vi "Prova QH.vi"(4 "solo acquisizione!!":bool=TRUE, 6 "Text.Text":string="Prova QH: ", 7 "Tipo motore pompa":enum16{"Monofase", "Trifase"}(ring), 8 "Array % valvole":dbl[][](array[numeric]), 9 "Manuale F\\auto T":bool=TRUE, 10 "Status":refnum<vi>, 11 "input cluster":T1={"Scelta wattmetro"={"Wattmetro"=enum."No Selection"}, "SET RPM"=0.0, "SET TEMP"=0.0, "Array banchi"=[{"Nome"="Elettropompa", "Tors. scala1"=0, "Tors. scala2"=0, "rpm"=0, "TAMB"=0, "Indici Temperature"=[0, 1], "Indice freno"=1, "alimentatore trifase"=0, "alimentatore monofase"=0, "alimentatore dc arm"=0, "alimentatore dc ecc"=0, "alimentatore dc mp"=0}, {"Nome"="Sommersa", "Tors. scala1"=0, "Tors. scala2"=0, "rpm"=0, "TAMB"=1, "Indici Temperature"=[0, 1], "Indice freno"=0, "alimentatore trifase"=0, "alimentatore monofase"=0, "alimentatore dc arm"=0, "alimentatore dc ecc"=0, "alimentatore dc mp"=0}], "Array valvole linee avvio/fermata"=[], "banco selezionato"=0, "Nomi valvole prop sistema"=[], "canale-- sensore"=[], "Attriti B1"=[], "Attriti B2"=[], "Collegamento elettrico"={"ALIMENTAZIONE ELETTRICA"=enum."AC MONOFASE", "ID"=0, "#rami freddo\\eq term resmeter"=0, "#rami riscaldamento resmeter"=0, "#rami freddo\\eq term resistomat"=0, "#rami riscaldamento resistomat"=0, "CALCOLI"=enum."AC TRIFASE"}, "lingua"=0, "Costanti collaudo"={"P [bar]"=0.0, "T amb. [°C]"=0.0, "Umidità [%]"=0.0, "T acqua [°C] 2"=0.0}, "OPZIONI MISURE RES"={"MISURA A FREDDO"=enum."RESISTOMAT", "MISURA EQ. TERMICO"=enum."RESISTOMAT", "MISURA DT PROVA IN CORSO"=enum."RESISTOMAT - CON FERMATE", "MISURE PRIMA E DOPO"=enum."RESISTOMAT", "STRUMENTI PRESENTI"=enum."NESSUNO"}, "Dati targa motore"={"Vnom"=0.0, "Fnom"=0.0, "Inom"=0.0, "Cnom"=0.0, "Npoli"=0.0, "Scorta 1"=0.0, "Scorta 2"=0.0, "Scorta 3"=0.0}}) -> ()   [LabVIEW 2019]
uses:
  Tstabilizzazione auto.vi
  SubVI ELETTROTEST60A Folder/Elettrotest60A/Global_bypass_ResMeter.vi
  TypeDef/WT SELECTION.ctl
  TypeDef/Definizione linea.ctl
  TypeDef/Cluster INFO.ctl
  TypeDef/Collegamenti_elettrici.ctl
  TypeDef/Control Calcoli.ctl
panel:
  out "Fine acq":bool
  in  "Reset":bool
  out "Set% valvole":dbl[](array[numeric])
  in  "Stato auto":string
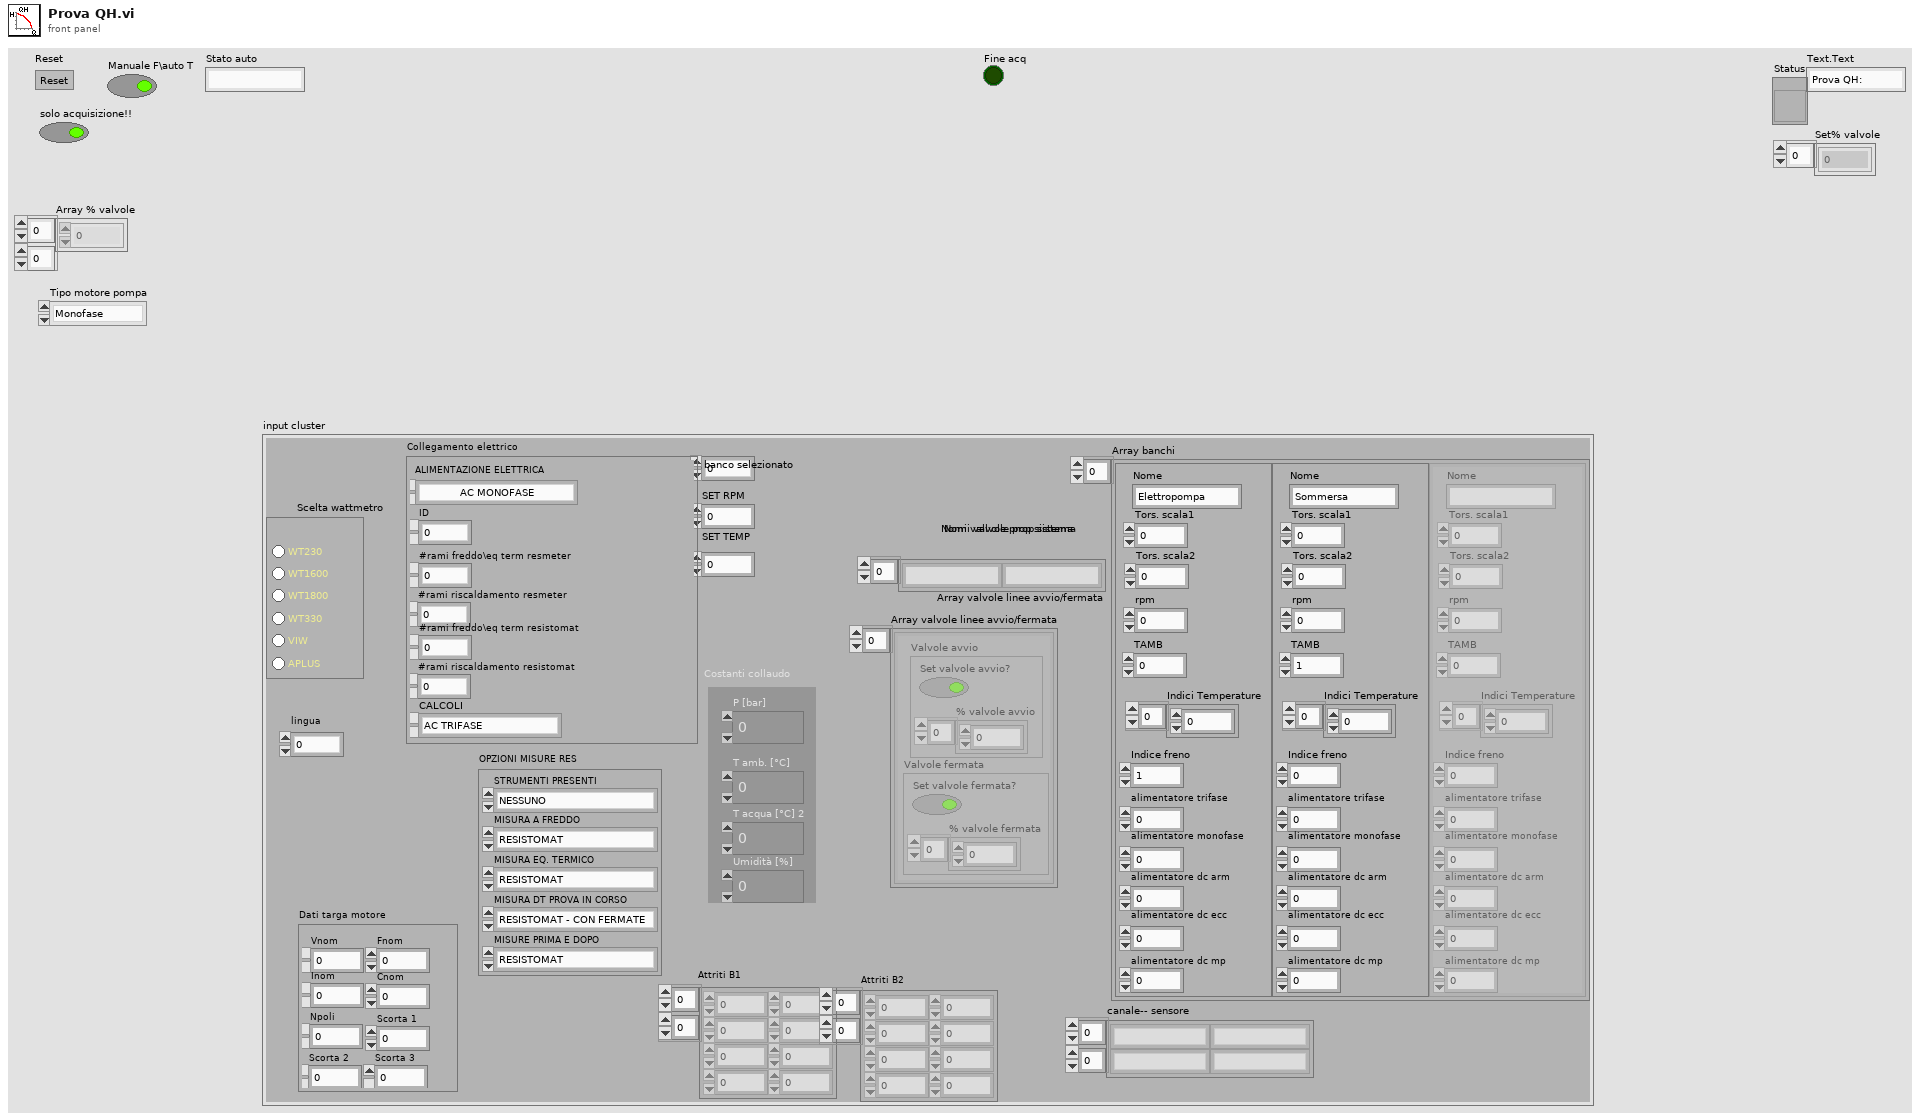
[diagram p1: front panel]
types:
  T1 = typedef "Cluster INFO.ctl" = cluster{"Scelta wattmetro":cluster{"Wattmetro":T2}, "SET RPM":dbl, "SET TEMP":dbl, "Array banchi":T3[], "Array valvole linee avvio/fermata":cluster{"Valvole avvio":cluster{"Set valvole avvio?":bool, "% valvole avvio":dbl[]}, "Valvole fermata":cluster{"Set valvole fermata?":bool, "% valvole fermata":dbl[]}}[], "banco selezionato":i8, "Nomi valvole prop sistema":string[], "canale-- sensore":string[][], "Attriti B1":dbl[][], "Attriti B2":dbl[][], "Collegamento elettrico":cluster{"ALIMENTAZIONE ELETTRICA":T4, "ID":i16, "#rami freddo\\eq term resmeter":i16, "#rami riscaldamento resmeter":i16, "#rami freddo\\eq term resistomat":i16, "#rami riscaldamento resistomat":i16, "CALCOLI":T5}, "lingua":i16, "Costanti collaudo":cluster{"P [bar]":dbl, "T amb. [°C]":dbl, "Umidità [%]":dbl, "T acqua [°C] 2":dbl}, "OPZIONI MISURE RES":cluster{"MISURA A FREDDO":enum16{"NESSUNO", "RESISTOMAT", "RES METER", "ENTRAMBI"}, "MISURA EQ. TERMICO":enum16{"NESSUNO", "RESISTOMAT", "RES METER", "ENTRAMBI"}, "MISURA DT PROVA IN CORSO":enum16{"NESSUNO", "RESISTOMAT - CON FERMATE", "RES METER - CON FERMATE", "RES METER - CONTINUO"}, "MISURE PRIMA E DOPO":enum16{"NESSUNO", "RESISTOMAT", "RES METER"}, "STRUMENTI PRESENTI":enum16{"NESSUNO", "RESISTOMAT", "RES METER", "ENTRAMBI"}}, "Dati targa motore":cluster{"Vnom":dbl, "Fnom":dbl, "Inom":dbl, "Cnom":dbl, "Npoli":dbl, "Scorta 1":dbl, "Scorta 2":dbl, "Scorta 3":dbl}}
  T2 = typedef "WT SELECTION.ctl" = enum32{"No Selection", "WT230", "WT1600", "WT1800", "WT330", "VIW", "APLUS"}
  T3 = typedef "Definizione linea.ctl" = cluster{"Nome":string, "Tors. scala1":i32, "Tors. scala2":i32, "rpm":i32, "TAMB":i32, "Indici Temperature":i16[], "Indice freno":i16, "alimentatore trifase":i16, "alimentatore monofase":i16, "alimentatore dc arm":i16, "alimentatore dc ecc":i16, "alimentatore dc mp":i16}
  T4 = typedef "Collegamenti_elettrici.ctl" = enum16{"AC TRIFASE", "AC TRIFASE + FRENO", "AC MONOFASE", "DC CON ECCITAZIONE", "DC CON ECCITAZIONE + FRENO", "DC NO ECCITAZIONE", "DC NO ECCITAZIONE + FRENO", "FRENO TRASC + AFE", "SOLO FRENO", "CARICO RESISTIVO", "GENERICO", "SOLO ACQUISITORE", "SCORTA 4", "SCORTA 5", "SCORTA 6"}
  T5 = typedef "Control Calcoli.ctl" = enum16{"AC TRIFASE", "AC MONOFASE", "DC ECCITAZIONE", "DC NO ECCITAZIONE", "POMPA TRIFASE", "POMPA MONOFASE", "GENERICO", "TRASFORMATORE", "ALTERNATORE TRASCINATO", "GRUPPO ELETTROGENO"}
  T6 = cluster{"Valvole avvio":cluster{"Set valvole avvio?":bool, "% valvole avvio":dbl[]}, "Valvole fermata":cluster{"Set valvole fermata?":bool, "% valvole fermata":dbl[]}}[]
  T7 = cluster{"Valvole avvio":cluster{"Set valvole avvio?":bool, "% valvole avvio":dbl[]}, "Valvole fermata":cluster{"Set valvole fermata?":bool, "% valvole fermata":dbl[]}}
  T8 = cluster{"Set valvole avvio?":bool, "% valvole avvio":dbl[]}
  T9 = cluster{"Set valvole fermata?":bool, "% valvole fermata":dbl[]}
  T10 = cluster{"Array of elements":cluster{"String":string, "variant":variant}[], "Single element":cluster{"String":string, "variant":variant}, "enque at\nopposite end (F)":bool, "no replications (F)":bool}
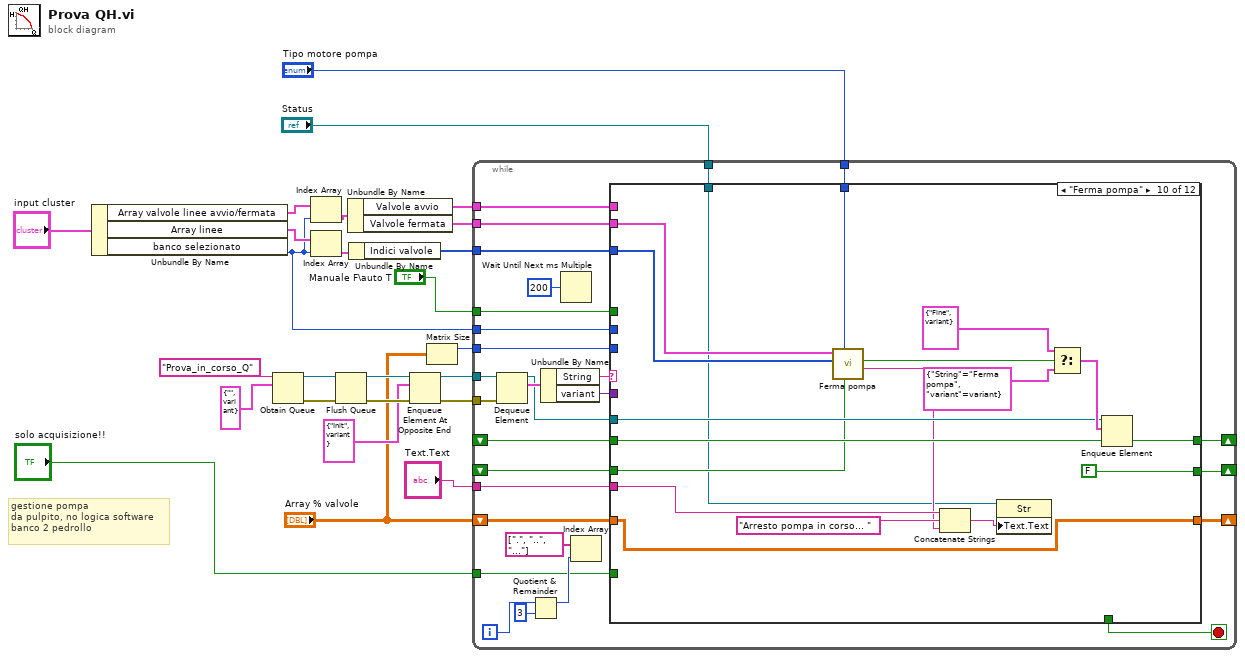
[diagram p0: block diagram]
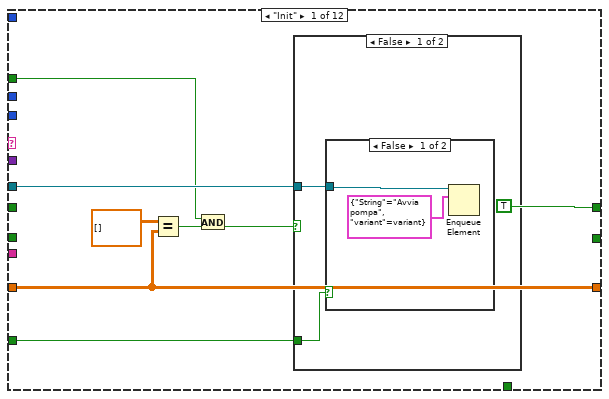
[diagram p2: hidden frame]
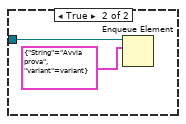
[diagram p3: hidden frame]
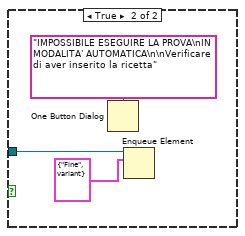
[diagram p4: hidden frame]
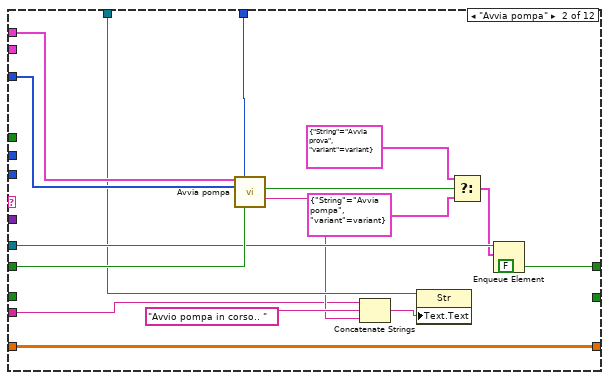
[diagram p5: hidden frame]
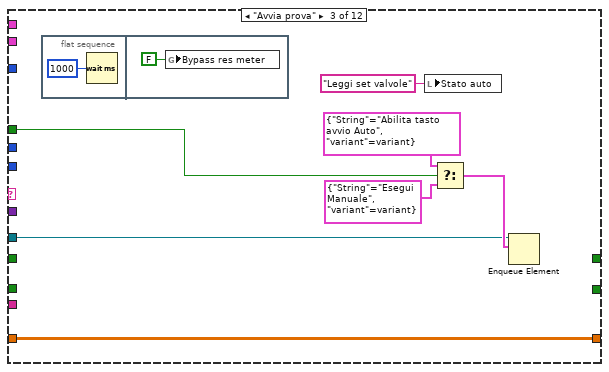
[diagram p6: hidden frame]
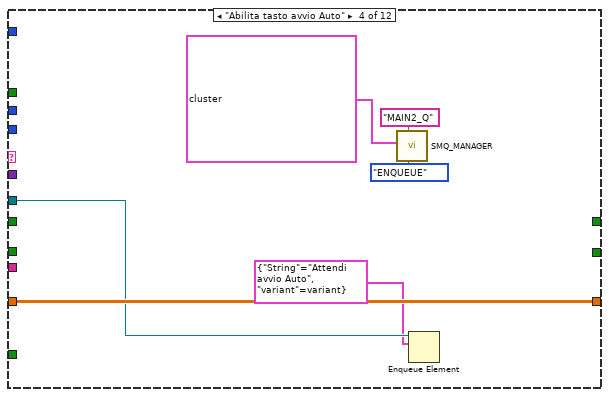
[diagram p7: hidden frame]
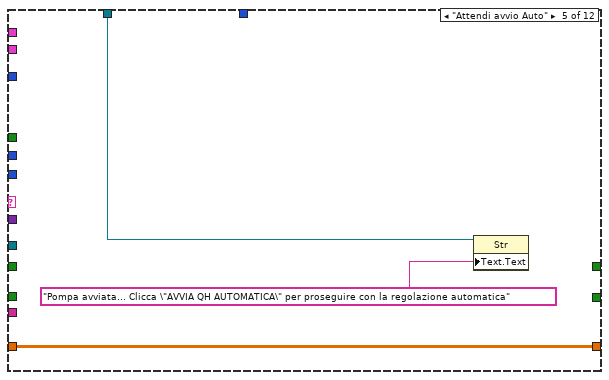
[diagram p8: hidden frame]
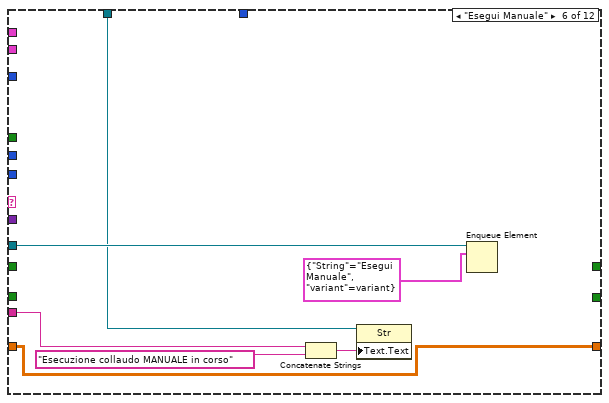
[diagram p9: hidden frame]
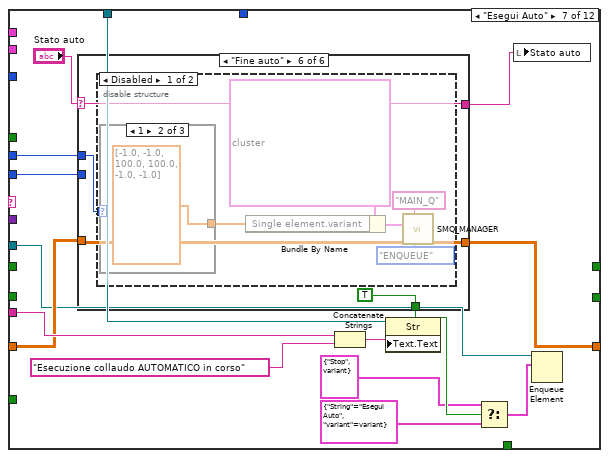
[diagram p10: hidden frame]
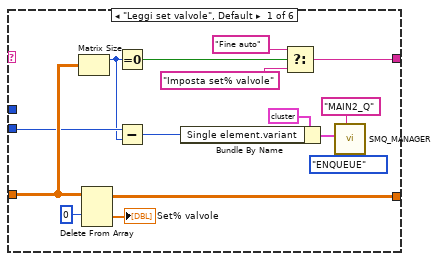
[diagram p11: hidden frame]
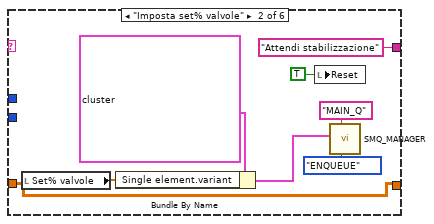
[diagram p12: hidden frame]
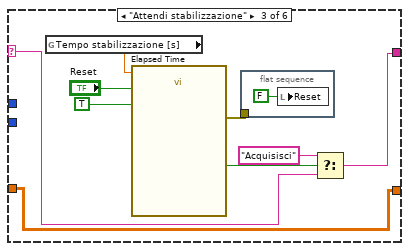
[diagram p13: hidden frame]
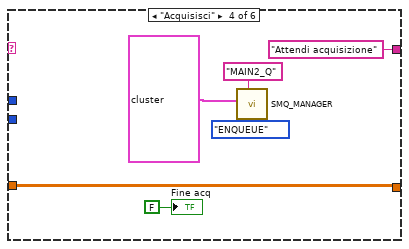
[diagram p14: hidden frame]
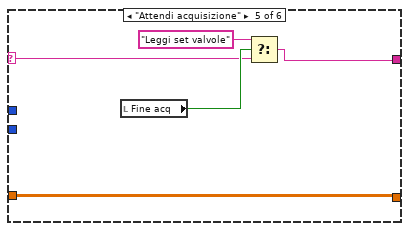
[diagram p15: hidden frame]
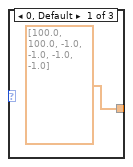
[diagram p16: hidden frame]
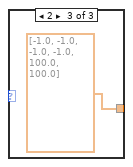
[diagram p17: hidden frame]
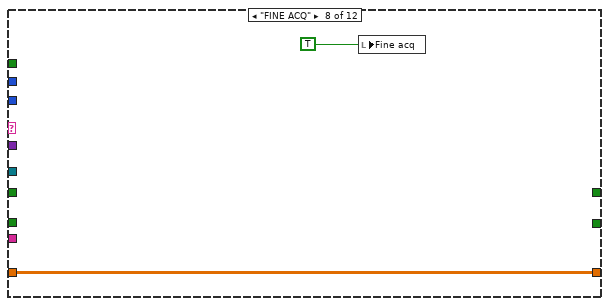
[diagram p19: hidden frame]
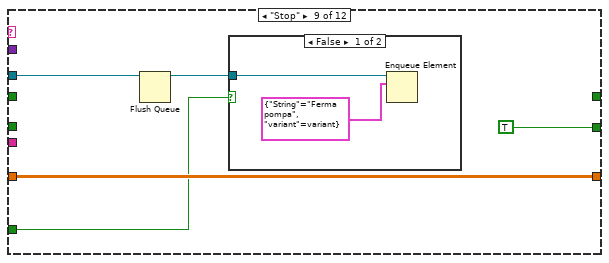
[diagram p20: hidden frame]
diagram:
  # "gestione pompa\nda pulpito, no logica software\nbanco 2 pedrollo"
  n1 = Unbundle By Name("input cluster") -> ("Array valvole linee avvio/fermata"=w12:T6, "Array linee"=w14:T3[], "banco selezionato"=w2:i8)
  n2 = Obtain Queue(name (unnamed)="Prova_in_corso_Q" ("Queue Name"), element data type=cluster{"String":string, "variant":variant} {"String"="", "variant"=variant} ("element")) -> (queue out=w19:refnum<queue>, error out=w18:errorcluster)  [unwired: 3 in, 1 out]
  n3 = Index Array(array=w12, index=w2) -> (element=w11:T7)
  n4 = Index Array(array=w14, index=w2) -> (element=w13:T3)
  n5 = Flush Queue(queue=w19, error in (no error)=w18) -> (queue out=w23:refnum<queue>, error out=w22:errorcluster)  [unwired: 1 out]
  n6 = Unbundle By Name(w11) -> ("Valvole avvio"=w9:T8, "Valvole fermata"=w8:T9)
  n7 = Unbundle By Name(w13) -> ("Indici valvole"=w7:i16[])
  n8 = Enqueue Element At Opposite End(queue=w23, element=cluster{"String":string, "variant":variant} {"String"="Init", "variant"=variant}, error in (no error)=w22) -> (queue out=w25:refnum<queue>, error out=w24:errorcluster)  [unwired: 1 in, 1 out]
  n9 = Matrix Size(0:"Array % valvole") -> (1:w3:i32)  [unwired: 1 out]
  n10 = while {
    tunnel: w25 -> [w53]
    tunnel: w24 -> [w52]
    tunnel: "Manuale F\\auto T" -> [w48]
    shift-right: [w47] -> _
    shift-left: "Array % valvole" -> [w46]
    shift-right: [w44] -> _
    shift-left: _ -> [w43]
    tunnel: w9 -> [w42]
    tunnel: "Tipo motore pompa" -> [w41]
    tunnel: w8 -> [w40]
    shift-right: [w39] -> _
    shift-left: _ -> [w38]
    tunnel: w7 -> [w37]
    tunnel: "Status" -> [w36]
    tunnel: "Text.Text" -> [w34]
    tunnel: w3 -> [w28]
    tunnel: "solo acquisizione!!" -> [w27]
    tunnel: w2 -> [w26]
    i -> [w30]
    stop <- w35 stop-if-true
    n11 = Dequeue Element(queue=w53, error in (no error)=w52) -> (queue out=w45:refnum<queue>, element=w51:cluster{"String":string, "variant":variant})  [unwired: 1 in, 2 out]
    n12 = Quotient & Remainder(x=w30, y=3) -> (x-y*floor(x/y)=w33:i32)  [unwired: 1 out]
    n13 = Unbundle By Name(w51) -> ("String"=w50:string, "variant"=w49:variant)
    n14 = Wait Until Next ms Multiple(millisecond multiple=u32 200) -> ()  [unwired: 1 out]
    n15 = Index Array(array=string[] [".", "..", "..."], index=w33) -> ()  [unwired: 1 out]
    n16 = case shown="\"Ferma pompa\"" w50 {
      selector: w50 -> [_ _ _ _ _ _ _ _ _ _ _ w216]
      tunnel: w49 -> [_ _ _ _ _ _ _ _ _ _ _ _]
      tunnel: w48 -> [w55 _ w89 _ _ _ _ _ _ _ _ _]
      tunnel: [w61 w79 w88 w101 w104 w105 w120 w185 w187 w195 w213 w217] -> w47
      tunnel: w46 -> [w61 w79 w88 w101 w104 w105 w121 w185 w187 w195 w213 w217]
      tunnel: w45 -> [w58 w84 w90 w100 _ w110 w118 _ w190 w204 _ _]
      tunnel: [TRUE FALSE _ _ _ _ _ _ _ w209 _ _] -> w44
      tunnel: w43 -> [_ w86 _ _ _ _ _ _ _ w209 _ _]
      tunnel: w42 -> [_ w77 _ _ _ _ _ _ _ _ _ _]
      tunnel: w41 -> [_ w78 _ _ _ _ _ _ _ w210 _ _]
      tunnel: w40 -> [_ _ _ _ _ _ _ _ _ w202 _ _]
      tunnel: [_ _ _ _ _ _ _ _ TRUE FALSE _ _] -> w39
      tunnel: w38 -> [_ _ _ _ _ _ _ _ _ w203 _ _]
      tunnel: w37 -> [_ w76 _ _ _ _ _ _ _ w201 _ _]
      tunnel: w36 -> [_ w75 _ _ w103 w109 w124 _ _ w196 _ _]
      tunnel: [_ _ _ _ _ _ _ _ _ _ TRUE _] -> w35
      tunnel: w34 -> [_ w71 _ _ _ w108 w123 _ _ w199 _ _]
      tunnel: w28 -> [_ _ _ _ _ _ w113 _ _ _ _ _]
      tunnel: w27 -> [w54 _ _ _ _ _ _ _ w186 _ _ _]
      tunnel: w26 -> [_ _ _ _ _ _ w112 _ _ _ _ _]
      frame "Init" {
        n17 = Equal?(x=dbl[][] [], y=w61) -> (x = y?=w59:bool)
        n18 = And(x=w55, y=w59) -> (x .and. y?=w56:bool)
        n19 = case shown="False" w56 {
          tunnel: w58 -> [w63 w69]
          tunnel: w54 -> [w62 _]
          frame False {
            n20 = case shown="False" w62 {
              tunnel: w63 -> [w64 w66]
              frame False {
                n21 = Enqueue Element(queue=w64, element=cluster{"String":string, "variant":variant} {"String"="Avvia pompa", "variant"=variant}) -> ()  [unwired: 2 in, 3 out]
              }
              frame True {
                n22 = Enqueue Element(queue=w66, element=cluster{"String":string, "variant":variant} {"String"="Avvia prova", "variant"=variant}) -> ()  [unwired: 2 in, 3 out]
              }
            }
          }
          frame True {
            n23 = One Button Dialog(message="IMPOSSIBILE ESEGUIRE LA PROVA\nIN MODALITA' AUTOMATICA\n\nVerificare di aver inserito la ricetta") -> ()  [unwired: 1 in, 1 out]
            n24 = Enqueue Element(queue=w69, element=cluster{"String":string, "variant":variant} {"String"="Fine", "variant"=variant}) -> ()  [unwired: 2 in, 3 out]
          }
        }
      }
      frame "Avvia pompa" {
        n25 = call "Avvia pompa.vi"("Valvole avvio"=w77, "Tipo motore pompa"=w78, "Indici valvole linea"=w76, "Reset avvio"=w86) -> ("Fine Avvio"=w83:bool, "stato"=w72:string)  [unwired: 10 in]
        n26 = Concatenate Strings(w71, "Avvio pompa in corso.. " ("Text.Text"), w72) -> (w73:string)
        n27 = property class="Str"(reference=w75, "Text.Text"=w73) -> ()  [unwired: 1 in, 2 out]
        n28 = Select(t=cluster{"String":string, "variant":variant} {"String"="Avvia prova", "variant"=variant} ("element"), s=w83, f=cluster{"String":string, "variant":variant} {"String"="Avvia pompa", "variant"=variant} ("element")) -> (s? t:f=w81:cluster{"String":string, "variant":variant})
        n29 = Enqueue Element(queue=w84, element=w81) -> ()  [unwired: 2 in, 3 out]
      }
      frame "Avvia prova" {
        n30 = flat-sequence {
          frame #0 {
            n31 = Wait (ms)(milliseconds to wait=u32 1000) -> ()  [unwired: 1 out]
          }
          frame #1 {
            n32 = global write "Global_bypass_ResMeter.vi" "Bypass res meter"(FALSE ("Bypass res meter")) -> ()
          }
        }
        n33 = local write "Stato auto"("Leggi set valvole" ("Stato auto")) -> ()
        n34 = Select(t=cluster{"String":string, "variant":variant} {"String"="Abilita tasto avvio Auto", "variant"=variant} ("element"), s=w89, f=cluster{"String":string, "variant":variant} {"String"="Esegui Manuale", "variant"=variant} ("element")) -> (s? t:f=w92:cluster{"String":string, "variant":variant})
        n35 = Enqueue Element(queue=w90, element=w92) -> ()  [unwired: 2 in, 3 out]
      }
      frame "Abilita tasto avvio Auto" {
        n36 = call <userlib>:"SMQ_MANAGER.vi"("Function"=enum16{"INITIALIZE", "ENQUEUE", "STOP ALL"}."ENQUEUE", "Queue name"="MAIN2_Q", "Enqueue cluster"=T10 {"Array of elements"=[], "Single element"={"String"="ABILITA TASTO AVVIO AUTO", "variant"=variant}, "enque at\nopposite end (F)"=FALSE, "no replications (F)"=FALSE}) -> ()  [unwired: 8 in, 1 out]
        n37 = Enqueue Element(queue=w100, element=cluster{"String":string, "variant":variant} {"String"="Attendi avvio Auto", "variant"=variant}) -> ()  [unwired: 2 in, 3 out]
      }
      frame "Attendi avvio Auto" {
        n38 = property class="Str"(reference=w103, "Text.Text"="Pompa avviata... Clicca \"AVVIA QH AUTOMATICA\" per proseguire con la regolazione automatica") -> ()  [unwired: 1 in, 2 out]
      }
      frame "Esegui Manuale" {
        n39 = Concatenate Strings(w108, "Esecuzione collaudo MANUALE in corso" ("string")) -> (w107:string)
        n40 = property class="Str"(reference=w109, "Text.Text"=w107) -> ()  [unwired: 1 in, 2 out]
        n41 = Enqueue Element(queue=w110, element=cluster{"String":string, "variant":variant} {"String"="Esegui Manuale", "variant"=variant}) -> ()  [unwired: 2 in, 3 out]
      }
      frame "Esegui Auto" {
        n42 = case shown="\"Fine auto\"" "Stato auto" {
          selector: "Stato auto" -> [_ _ w153 _ w169 w174]
          tunnel: w121 -> [w138 w142 w150 w160 w166 w173]
          tunnel: [w140 w142 w150 w160 w166 w173] -> w120
          tunnel: [w135 "Attendi stabilizzazione" w152 "Attendi acquisizione" ("t") w168 w174] -> w119
          tunnel: [_ _ _ _ _ TRUE] -> w115
          tunnel: w113 -> [w133 _ _ _ _ _]
          tunnel: w112 -> [_ _ _ _ _ w172]
          frame "Leggi set valvole", Default {
            n43 = Matrix Size(0:w138) -> (1:w132:i32)  [unwired: 1 out]
            n44 = Delete From Array(array=w138, index (row)=0) -> (deleted portion=→"Set% valvole":dbl[], array with subset deleted=w140:dbl[][])  [unwired: 2 in]
            n45 = Equal To 0?(x=w132) -> (x = 0?=w137:bool)
            n46 = Subtract(x=w133, y=w132) -> (x-y=w127:i32)
            n47 = Bundle By Name(cluster=T10 {"Array of elements"=[], "Single element"={"String"="PUNTO QH AUTO", "variant"=variant}, "enque at\nopposite end (F)"=FALSE, "no replications (F)"=FALSE} ("Enqueue cluster"), "Single element.variant"=w127) -> (w131:T10)
            n48 = Select(t="Fine auto", s=w137, f="Imposta set% valvole") -> (s? t:f=w135:string)
            n49 = call <userlib>:"SMQ_MANAGER.vi"("Function"=enum16{"INITIALIZE", "ENQUEUE", "STOP ALL"}."ENQUEUE", "Queue name"="MAIN2_Q", "Enqueue cluster"=w131) -> ()  [unwired: 8 in, 1 out]
          }
          frame "Imposta set% valvole" {
            n50 = local read "Set% valvole"() -> (w145:dbl[])
            n51 = Bundle By Name(cluster=T10 {"Array of elements"=[], "Single element"={"String"="COMANDI VALVOLE PROP", "variant"=variant}, "enque at\nopposite end (F)"=FALSE, "no replications (F)"=FALSE} ("Enqueue cluster"), "Single element.variant"=w145) -> (w149:T10)
            n52 = local write "Reset"(TRUE ("Reset")) -> ()
            n53 = call <userlib>:"SMQ_MANAGER.vi"("Function"=enum16{"INITIALIZE", "ENQUEUE", "STOP ALL"}."ENQUEUE", "Queue name"="MAIN_Q", "Enqueue cluster"=w149) -> ()  [unwired: 8 in, 1 out]
          }
          frame "Attendi stabilizzazione" {
            n54 = global read "Tstabilizzazione auto.vi" "Tempo stabilizzazione [s]"() -> (w155:dbl)
            n55 = call "Elapsed Time"("Time Target (s)"=w155, "Reset"="Reset", "Auto Reset"=TRUE) -> ("Time has Elapsed"=w154:bool, "error out"=w156:errorcluster)  [unwired: 9 in, 6 out]
            n56 = flat-sequence {
              tunnel: w156 -> [_]
              frame #0 {
                n57 = local write "Reset"(FALSE ("Reset")) -> ()
              }
            }
            n58 = Select(t="Acquisisci", s=w154, f=w153) -> (s? t:f=w152:string)
          }
          frame "Acquisisci" {
            n59 = call <userlib>:"SMQ_MANAGER.vi"("Function"=enum16{"INITIALIZE", "ENQUEUE", "STOP ALL"}."ENQUEUE", "Queue name"="MAIN2_Q", "Enqueue cluster"=T10 {"Array of elements"=[], "Single element"={"String"="AQ AUTO", "variant"=variant}, "enque at\nopposite end (F)"=FALSE, "no replications (F)"=FALSE}) -> ()  [unwired: 8 in, 1 out]
            "Fine acq" <- FALSE
          }
          frame "Attendi acquisizione" {
            n60 = local read "Fine acq"() -> (w170:bool)
            n61 = Select(t="Leggi set valvole", s=w170, f=w169) -> (s? t:f=w168:string)
          }
          frame "Fine auto" {
            n62 = disable-structure shown="Disabled" {
              disable-tunnel: w172 -> [w176 _]
              frame Disabled {
                n63 = case shown="1" w176 {
                  tunnel: [dbl[] [100.0, 100.0, -1.0, -1.0, -1.0, -1.0] dbl[] [-1.0, -1.0, 100.0, 100.0, -1.0, -1.0] dbl[] [-1.0, -1.0, -1.0, -1.0, 100.0, 100.0]] -> w175
                  frame 0, Default {
                  }
                  frame 1 {
                  }
                  frame 2 {
                  }
                }
                n64 = Bundle By Name(cluster=T10 {"Array of elements"=[], "Single element"={"String"="COMANDI VALVOLE PROP", "variant"=variant}, "enque at\nopposite end (F)"=FALSE, "no replications (F)"=FALSE} ("Enqueue cluster"), "Single element.variant"=w175) -> (w180:T10)
                n65 = call <userlib>:"SMQ_MANAGER.vi"("Function"=enum16{"INITIALIZE", "ENQUEUE", "STOP ALL"}."ENQUEUE", "Queue name"="MAIN_Q", "Enqueue cluster"=w180) -> ()  [unwired: 8 in, 1 out]
              }
              frame Enabled {
              }
            }
          }
        }
        n66 = Concatenate Strings(w123, "Esecuzione collaudo AUTOMATICO in corso" ("string")) -> (w126:string)
        n67 = property class="Str"(reference=w124, "Text.Text"=w126) -> ()  [unwired: 1 in, 2 out]
        n68 = Select(t=cluster{"String":string, "variant":variant} {"String"="Stop", "variant"=variant} ("element"), s=w115, f=cluster{"String":string, "variant":variant} {"String"="Esegui Auto", "variant"=variant} ("element")) -> (s? t:f=w116:cluster{"String":string, "variant":variant})
        n69 = local write "Stato auto"(w119) -> ()
        n70 = Enqueue Element(queue=w118, element=w116) -> ()  [unwired: 2 in, 3 out]
      }
      frame "FINE ACQ" {
        n71 = local write "Fine acq"(TRUE ("Fine acq")) -> ()
      }
      frame "Stop" {
        n72 = Flush Queue(queue=w190) -> (queue out=w189:refnum<queue>)  [unwired: 1 in, 2 out]
        n73 = case shown="False" w186 {
          tunnel: w189 -> [w191 w193]
          frame False {
            n74 = Enqueue Element(queue=w191, element=cluster{"String":string, "variant":variant} {"String"="Ferma pompa", "variant"=variant}) -> ()  [unwired: 2 in, 3 out]
          }
          frame True {
            n75 = Enqueue Element(queue=w193, element=cluster{"String":string, "variant":variant} {"String"="Fine", "variant"=variant}) -> ()  [unwired: 2 in, 3 out]
          }
        }
      }
      frame "Ferma pompa" {
        n76 = call "Ferma pompa.vi"("Reset fermata"=w203, "Tipo motore pompa"=w210, "Indici valvole linea"=w201, "Valvole fermata"=w202) -> ("stato"=w197:string, "Fine Fermata"=w205:bool)  [unwired: 6 in]
        n77 = Concatenate Strings(w199, "Arresto pompa in corso... " ("string"), w197) -> (w200:string)
        n78 = property class="Str"(reference=w196, "Text.Text"=w200) -> ()  [unwired: 1 in, 2 out]
        n79 = Select(t=cluster{"String":string, "variant":variant} {"String"="Fine", "variant"=variant} ("element"), s=w205, f=cluster{"String":string, "variant":variant} {"String"="Ferma pompa", "variant"=variant} ("element")) -> (s? t:f=w207:cluster{"String":string, "variant":variant})
        n80 = Enqueue Element(queue=w204, element=w207) -> ()  [unwired: 2 in, 3 out]
      }
      frame "Fine" {
      }
      frame "CASE INESISTENTE", Default {
        n81 = Concatenate Strings(w216, " CASE INESISTENTE" ("string")) -> (w215:string)
        n82 = One Button Dialog(message=w215) -> ()  [unwired: 1 in, 1 out]
      }
    }
  }
